vi "PID.vi"(0 "Setpoint":dbl, 1 "PID Gains":cluster{"Kp":dbl, "Ki":dbl, "Kd":dbl}, 2 "Process Variable":dbl, 3 "Reset":bool, 4 "dt (ms)":i64, 5 "Min/Max Controlable Values":T1) -> (7 "Output":dbl)   [LabVIEW 2019]
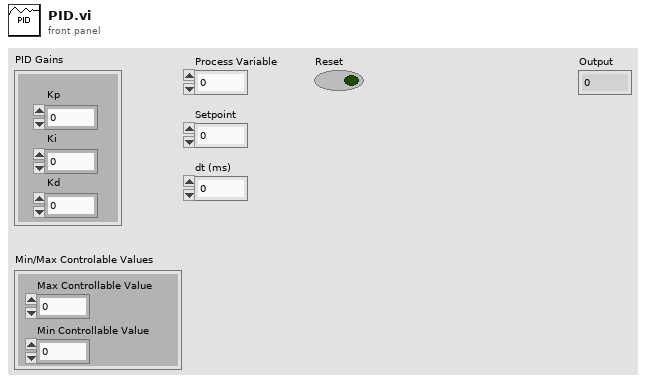
[diagram p1: front panel]
types:
  T1 = cluster{"Max Controllable Value":dbl, "Min Controllable Value":dbl}
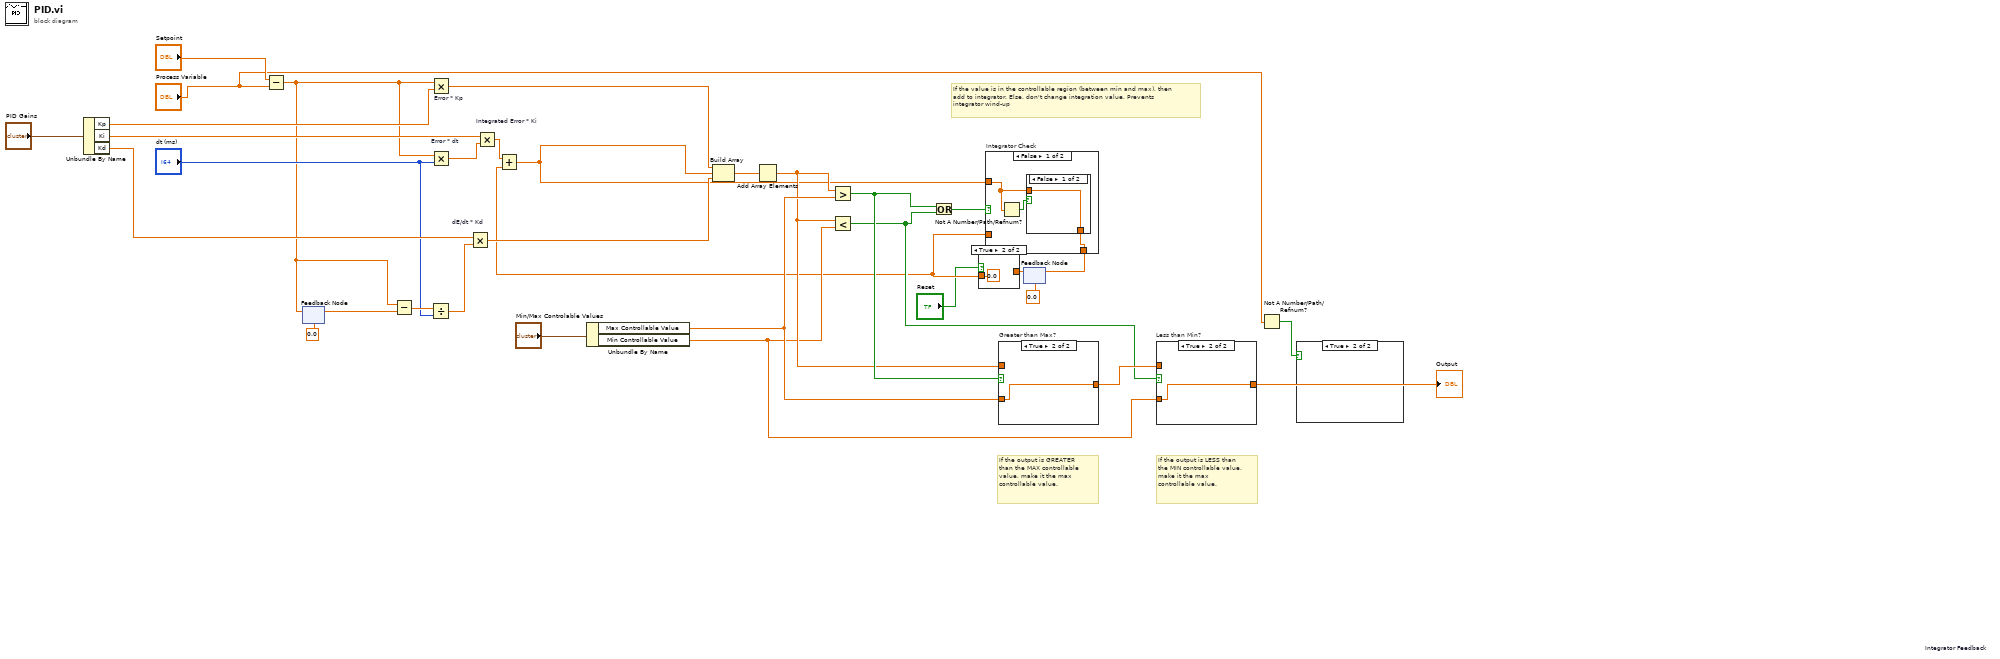
[diagram p0: block diagram]
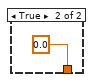
[diagram p6: hidden frame]
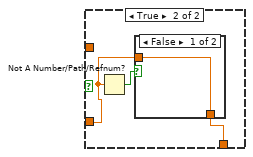
[diagram p7: hidden frame]
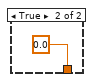
[diagram p8: hidden frame]
diagram:
  # "If the output is LESS than the MIN controllable value, make it the max controllable value."
  # "If the output is GREATER than the MAX controllable value, make it the max controllable value."
  # "If the value is in the controllable region (between min and max), then add to integrator. Else, don't change integration value. Prevents integrator wind-up"
  n1 = Unbundle By Name("PID Gains") -> ("Kp"=w31:dbl, "Ki"=w29:dbl, "Kd"=w28:dbl)
  n2 = Subtract(x="Setpoint", y="Process Variable") -> (x-y=w14:dbl)
  n3 = feedback-in #1(w14) -> ()
  n4 = feedback #1(0.0) -> (w15:dbl)
  n5 = Subtract(x=w14, y=w15) -> (x-y=w27:dbl)
  n6 = Divide(x=w27, y="dt (ms)") -> (x/y=w25:dbl)
  n7 = Multiply "Error * Kp"(x=w14, y=w31) -> (x*y=w22:dbl)
  n8 = Multiply "Error * dt"(x=w14, y="dt (ms)") -> (x*y=w6:dbl)
  n9 = Multiply "dE/dt * Kd"(x=w28, y=w25) -> (x*y=w21:dbl)
  n10 = Multiply "Integrated Error * Ki"(x=w29, y=w6) -> (x*y=w7:dbl)
  n11 = Unbundle By Name("Min/Max Controlable Values") -> ("Max Controllable Value"=w16:dbl, "Min Controllable Value"=w10:dbl)
  n12 = feedback #2 "Integrator Feedback"(0.0) -> (w5:dbl)
  n13 = case shown="True" "Reset" {
    tunnel: w5 -> [w34 _]
    tunnel: [w34 0.0] -> w4
    frame False {
    }
    frame True {
    }
  }
  n14 = Add(x=w7, y=w4) -> (x+y=w8:dbl)
  n15 = Build Array(w22, w8, w21) -> (w23:dbl[])
  n16 = Add Array Elements(numeric array=w23) -> (sum=w13:dbl)
  n17 = Greater?(x=w13, y=w16) -> (0:w17:bool)
  n18 = Less?(x=w13, y=w10) -> (x < y?=w11:bool)
  n19 = Or(x=w17, y=w11) -> (x .or. y?=w20:bool)
  n20 = case "Integrator Check" shown="False" w20 {
    tunnel: w8 -> [w37 _]
    tunnel: [w36 w41] -> w19
    tunnel: w4 -> [_ w42]
    frame False {
      n21 = Not A Number/Path/Refnum?(number/path/refnum=w37) -> (NaN/Path/Refnum?=w38:bool)
      n22 = case shown="False" w38 {
        tunnel: w37 -> [w39 _]
        tunnel: [w39 0.0] -> w36
        frame False {
        }
        frame True {
        }
      }
    }
    frame True {
      n23 = Not A Number/Path/Refnum?(number/path/refnum=w42) -> (NaN/Path/Refnum?=w43:bool)
      n24 = case shown="False" w43 {
        tunnel: w42 -> [w44 _]
        tunnel: [w44 0.0] -> w41
        frame False {
        }
        frame True {
        }
      }
    }
  }
  n25 = case "Greater than Max?" shown="True" w17 {
    tunnel: w13 -> [w46 _]
    tunnel: w16 -> [_ w47]
    tunnel: [w46 w47] -> w12
    frame False {
    }
    frame True {
    }
  }
  n26 = feedback-in #2(w19) -> ()
  n27 = case "Less than Min?" shown="True" w11 {
    tunnel: w12 -> [w48 _]
    tunnel: w10 -> [_ w49]
    tunnel: [w48 w49] -> w9
    frame False {
    }
    frame True {
    }
  }
  "Output" <- w9
  n28 = Not A Number/Path/Refnum?(number/path/refnum="Process Variable") -> (NaN/Path/Refnum?=w2:bool)
  n29 = case shown="True" w2 {
    frame False {
    }
    frame True {
    }
  }
